vi "Read Allowable Pairing Distances.vi"(8 "error in (no error)":errorcluster, 11 "E2E editor node in":refnum<data-value>) -> (0 "error out":errorcluster, 2 "Allowable Pairing Distances":i32[](array[numeric]), 3 "E2E editor node out":refnum<data-value>)   [LabVIEW 2015, in "E2E Tag Exchange editor node.lvclass"]
uses:
  E2E Tag Exchange editor node.lvclass
  module/configuration/E2E Tag Exchange configuration.lvclass
  module/configuration/E2E Tag Exchange configuration.lvclass/E2E Tag Exchange configuration.ctl
  <vilib>/NI/Configuration Framework/serializable configuration/NISE_CEF_serializable configuration.lvclass
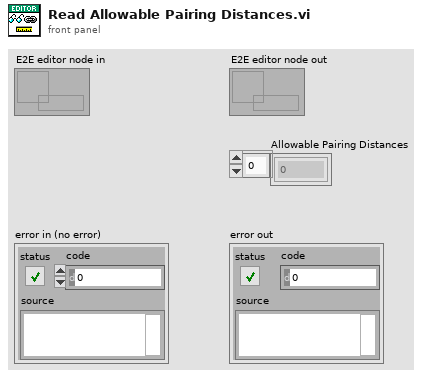
[diagram p1: front panel]
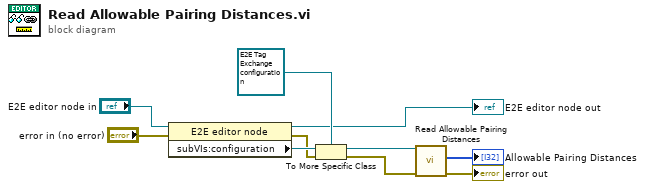
[diagram p0: block diagram]
diagram:
  n1 = property class="E2E editor node"(reference="E2E editor node in", error in="error in (no error)") -> (reference out=→"E2E editor node out":refnum<data-value>, error out=w8:errorcluster, "subVIs:configuration"=w9:refnum<class "NISE_CEF_serializable configuration.lvclass">)
  n2 = To More Specific Class(target class=refnum<class "E2E Tag Exchange configuration.lvclass"> refnum ("E2E configuration"), reference=w9, error in=w8) -> (specific class reference=w6:refnum<class "E2E Tag Exchange configuration.lvclass">, error out=w3:errorcluster)
  n3 = call "Read Allowable Pairing Distances.vi"("error in (no error)"=w3, "E2E configuration in"=w6) -> ("error out"=→"error out":errorcluster, "Allowable Pairing Distances"=→"Allowable Pairing Distances":i32[])  [unwired: 7 in, 1 out]
